vi "Hide VI Panel.vi"(8 "error in (no error)":errorcluster, 11 "VI":refnum<vi>) -> (0 "error out":errorcluster)   [LabVIEW 2020, in "Module 1.lvlib"]
doc: "Hide the panel of the specified VI.\n_____\nBased on DQMH Project Template 6.0.0.91."
uses:
  Module 1.lvlib
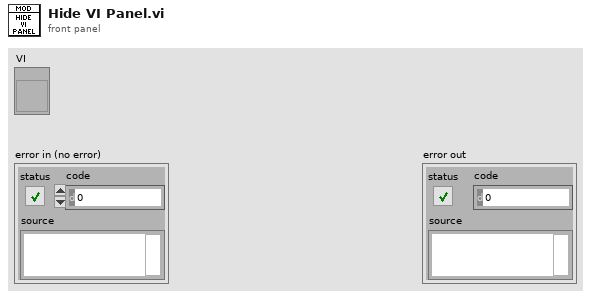
[diagram p1: front panel]
types:
  T1 = enum32{"Invalid", "Standard", "Closed", "Hidden", "Minimized", "Maximized"}
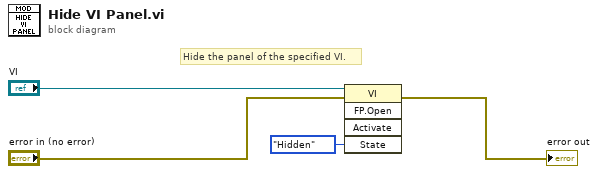
[diagram p0: block diagram]
diagram:
  # "Hide the panel of the specified VI."
  n1 = invoke class="VI" method="FP.Open"(reference="VI", error in="error in (no error)", "State"=T1."Hidden") -> (error out=→"error out":errorcluster)  [unwired: 2 in, 4 out]
